vi "CreateCircle.vi"(8 "Error In":errorcluster, 9 "r":dbl, 10 "Color":u32(colorbox)) -> (0 "Error Out":errorcluster, 3 "Circle out":refnum<class "Circle.lvclass">)   [LabVIEW 2021, in "Circle.lvclass"]
doc: "Create a object of cricle class."
uses:
  Circle.lvclass
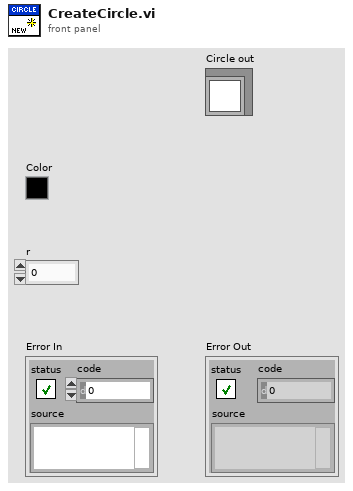
[diagram p1: front panel]
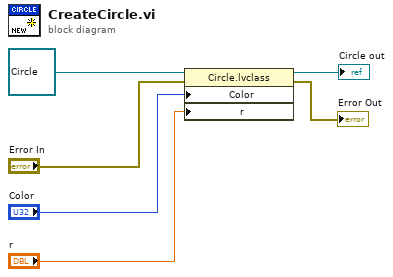
[diagram p0: block diagram]
diagram:
  n1 = property class="Circle.lvclass"(reference=refnum<class "Circle.lvclass"> refnum ("Circle in"), error in="Error In", "Color"="Color", "r"="r") -> (reference out=→"Circle out":refnum<class "Circle.lvclass">, error out=→"Error Out":errorcluster)
